vi "ultrasonic.vi"   [LabVIEW 2012, in "sumobot 18.lvrbt"]
uses:
  sumobot 18.lvrbt
  <vilib>/NXT/Block Support/NXT_OutputPort.ctl
  <vilib>/NXT/Block Support/NXT_InputPort.ctl
  <vilib>/NXT/Dual Mode Library/Sound/PlayRedPianoFile.vi
  <vilib>/NXT/Dual Mode Library/Waits/Wait_Num.vi
  <vilib>/NXT/NXTIO Xnodes/NXTIONodeSubVIs/NXTMoveMotors.vi
  <vilib>/NXT/NXTIO Xnodes/NXTIONodeSubVIs/LEGOStopAllMotors.vi
  <vilib>/NXT/Dual Mode Library/Sound/PlayB.vi
  <vilib>/NXT/Dual Mode Library/Sensors/Sonar_cm.vi
  <vilib>/NXT/Dual Mode Library/Sound/PlayC.vi
  <vilib>/NXT/Dual Mode Library/Sensors/Light_On.vi
  <vilib>/NXT/Dual Mode Library/Sound/PlayF.vi
  <vilib>/NXT/NXTIO Xnodes/NXTIONodeSubVIs/NXTStopMotors.vi
  <vilib>/NXT/NXTIO Xnodes/AddressXNode/NXTIOAddress.xnode
  <vilib>/NXT/NXTIO Xnodes/NXTIOXNode/NXTIO.xnode
  <vilib>/NXT/Subs/LVHSConnector.ctl
  <vilib>/NXT/LegoClasses/BrickReference/BrickReference.lvclass
types:
  T1 = typedef "LVHSConnector.ctl" = refnum<class "BrickReference.lvclass">
  T2 = typedef "NXT_OutputPort.ctl" = u8
  T3 = cluster{"Output Port":T2, "Output Port 2":T2, "Output Port 3":T2}
  T4 = typedef "NXT_InputPort.ctl" = u32
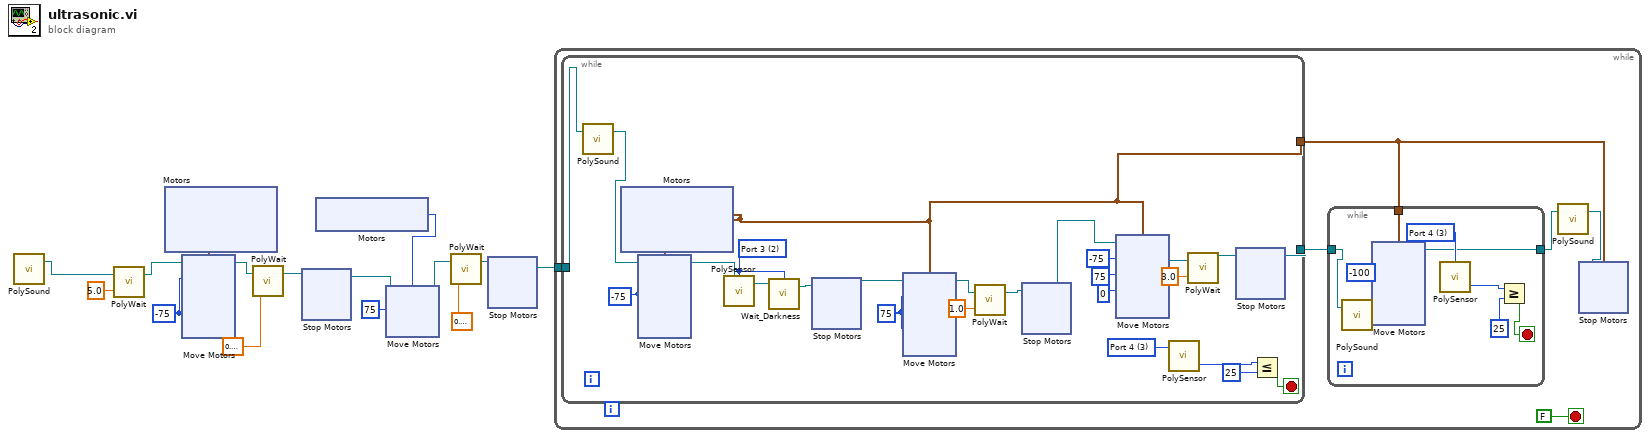
[diagram p0: block diagram]
diagram:
  w14 = i8 -75 ("Power/Speed 3")
  n1 = call-poly <vilib>:"PolySound.vi"() -> ("NXT/EV3"=w1:T1)  [unwired: 4 in]
  n2 = call-poly <vilib>:"PolyWait.vi"("Time (1 sec)"=sgl 5.0, "NXT/EV3"=w1) -> ("NXT/EV3"=w2:T1)  [unwired: 2 in]
  n3 = xnode "Motors"() -> ("Motor"=w8:cluster{"Port":T2, "Port":T2, "Port":T2})
  n4 = xnode "Move Motors"("Power/Speed 3"=w14, "Power/Speed 2"=w14, "Power/Speed 1"=w14, "Motors"=w8, "NXT/EV3"=w2) -> ("NXT/EV3"=w10:T1)
  n5 = call-poly <vilib>:"PolyWait.vi"("Time (1 sec)"=sgl 0.3, "NXT/EV3"=w10) -> ("NXT/EV3"=w12:T1)  [unwired: 2 in]
  n6 = xnode "Stop Motors"("NXT/EV3"=w12) -> ("NXT/EV3"=w13:T1)  [unwired: 1 in]
  n7 = xnode "Motors"() -> ("Motor"=w7:T2)
  n8 = xnode "Move Motors"("Power/Speed 1"=i8 75, "Motors"=w7, "NXT/EV3"=w13) -> ("NXT/EV3"=w3:T1)
  n9 = call-poly <vilib>:"PolyWait.vi"("Time (1 sec)"=sgl 0.2, "NXT/EV3"=w3) -> ("NXT/EV3"=w6:T1)  [unwired: 2 in]
  n10 = xnode "Stop Motors"("NXT/EV3"=w6) -> ("NXT/EV3"=w4:T1)  [unwired: 1 in]
  n11 = while {
    tunnel: w4 -> [w18]
    stop <- FALSE stop-if-true
    n12 = while {
      tunnel: [w53] -> w20
      tunnel: [w54] -> w21
      tunnel: w18 -> [w46]
      stop <- w56 stop-if-true
      w58 = T4 3 items=["Port 1", "Port 2", "Port 3", "Port 4"] ("Port (Port 4)")
      w49 = i8 -75 ("Power/Speed 2")
      w52 = i8 75 ("Power/Speed 2")
      w48 = T4 2 items=["Port 1", "Port 2", "Port 3", "Port 4"] ("Port (Port 3)")
      n13 = call-poly <vilib>:"PolySound.vi"("NXT/EV3"=w46) -> ("NXT/EV3"=w45:T1)  [unwired: 3 in]
      n14 = xnode "Motors"() -> ("Motor"=w53:cluster{"Port":T2, "Port":T2, "Port":T2})
      n15 = xnode "Move Motors"("Power/Speed 1"=w49, "Motors"=w53, "NXT/EV3"=w45, "Power/Speed 3"=w49, "Power/Speed 2"=w49) -> ("NXT/EV3"=w64:T1)
      n16 = call-poly <vilib>:"PolySensor.vi"("NXT/EV3"=w64, "Port (Port 3)"=w48) -> ("NXT/EV3"=w47:T1)  [unwired: 1 in, 1 out]
      n17 = call <vilib>:"Wait_Darkness.vi"("NXT/EV3"=w47, "Port (Port 3)"=w48) -> ("NXT/EV3"=w69:T1)  [unwired: 2 in]
      n18 = xnode "Stop Motors"("NXT/EV3"=w69) -> ("NXT/EV3"=w68:T1)  [unwired: 1 in]
      n19 = xnode "Move Motors"("Power/Speed 3"=w52, "Power/Speed 2"=w52, "Power/Speed 1"=w52, "Motors"=w53, "NXT/EV3"=w68) -> ("NXT/EV3"=w67:T1)
      n20 = call-poly <vilib>:"PolyWait.vi"("Time (1 sec)"=sgl 1.0, "NXT/EV3"=w67) -> ("NXT/EV3"=w65:T1)  [unwired: 2 in]
      n21 = xnode "Stop Motors"("NXT/EV3"=w65) -> ("NXT/EV3"=w62:T1)  [unwired: 1 in]
      n22 = xnode "Move Motors"("Power/Speed 3"=i8 0, "Power/Speed 2"=i8 75, "Power/Speed 1"=i8 -75, "Motors"=w53, "NXT/EV3"=w62) -> ("NXT/EV3"=w61:T1)
      n23 = call-poly <vilib>:"PolySensor.vi"("Port (Port 4)"=w58) -> ("Distance (cm)"=w55:i16)  [unwired: 2 in, 1 out]
      n24 = call-poly <vilib>:"PolyWait.vi"("Time (1 sec)"=sgl 3.0, "NXT/EV3"=w61) -> ("NXT/EV3"=w59:T1)  [unwired: 2 in]
      n25 = xnode "Stop Motors"("NXT/EV3"=w59) -> ("NXT/EV3"=w54:T1)  [unwired: 1 in]
      n26 = Less Or Equal?(x=w55, y=i16 25) -> (x <= y?=w56:bool)
    }
    n27 = while {
      tunnel: w20 -> [w35]
      tunnel: [w31] -> w17
      tunnel: w21 -> [w27]
      stop <- w30 stop-if-true
      w34 = T4 3 items=["Port 1", "Port 2", "Port 3", "Port 4"] ("Port (Port 4)")
      w29 = i8 -100 ("Power/Speed 2")
      n28 = call-poly <vilib>:"PolySound.vi"("NXT/EV3"=w27) -> ("NXT/EV3"=w28:T1)  [unwired: 3 in]
      n29 = xnode "Move Motors"("Power/Speed 3"=w29, "Power/Speed 2"=w29, "Power/Speed 1"=w29, "Motors"=w35, "NXT/EV3"=w28) -> ("NXT/EV3"=w31:T1)
      n30 = call-poly <vilib>:"PolySensor.vi"("Port (Port 4)"=w34) -> ("Distance (cm)"=w33:i16)  [unwired: 2 in, 1 out]
      n31 = Greater Or Equal?(x=w33, y=25) -> (x >= y?=w30:bool)
    }
    n32 = call-poly <vilib>:"PolySound.vi"("NXT/EV3"=w17) -> ("NXT/EV3"=w16:T1)  [unwired: 3 in]
    n33 = xnode "Stop Motors"("Motors"=w20, "NXT/EV3"=w16) -> ()  [unwired: 1 out]
  }
